vi "Temp Fuel Gen.vi"() -> ()   [LabVIEW 2017]
uses:
  Type defs/Control 1.ctl
panel:
  in  "f_q":dbl[][](array[numeric])
  in  "temp typedef":dbl[][](array[numeric])
  in  "Avg fuel 2":T1
  in  "output cluster 2":T1
  in  "Miliseconds to wait":dbl=1000.0 min=1000.0 step=1.0
  in  "Tryb auto":bool
  in  "Exit":bool
  in  "Wygeneruj":bool
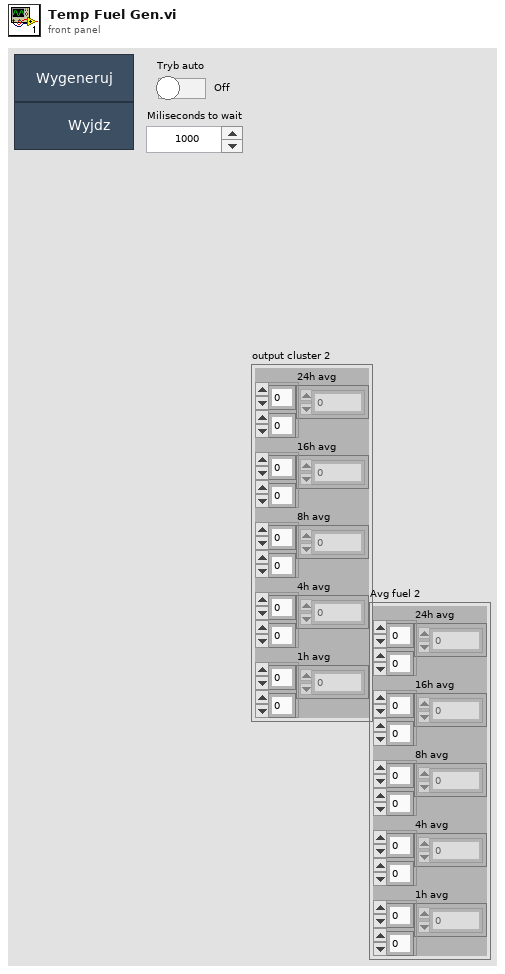
[diagram p1: front panel]
types:
  T1 = cluster{"24h avg":dbl[][], "16h avg":dbl[][], "8h avg":dbl[][], "4h avg":dbl[][], "1h avg":dbl[][]}
  T2 = typedef "Control 1.ctl" = enum16{"generate", "generate2", "wait for input", "timeout", "exit"}
  T3 = cluster{"Array":dbl[][], "Array":dbl[][], "Array":dbl[][], "Array":dbl[][], "Array":dbl[][]}
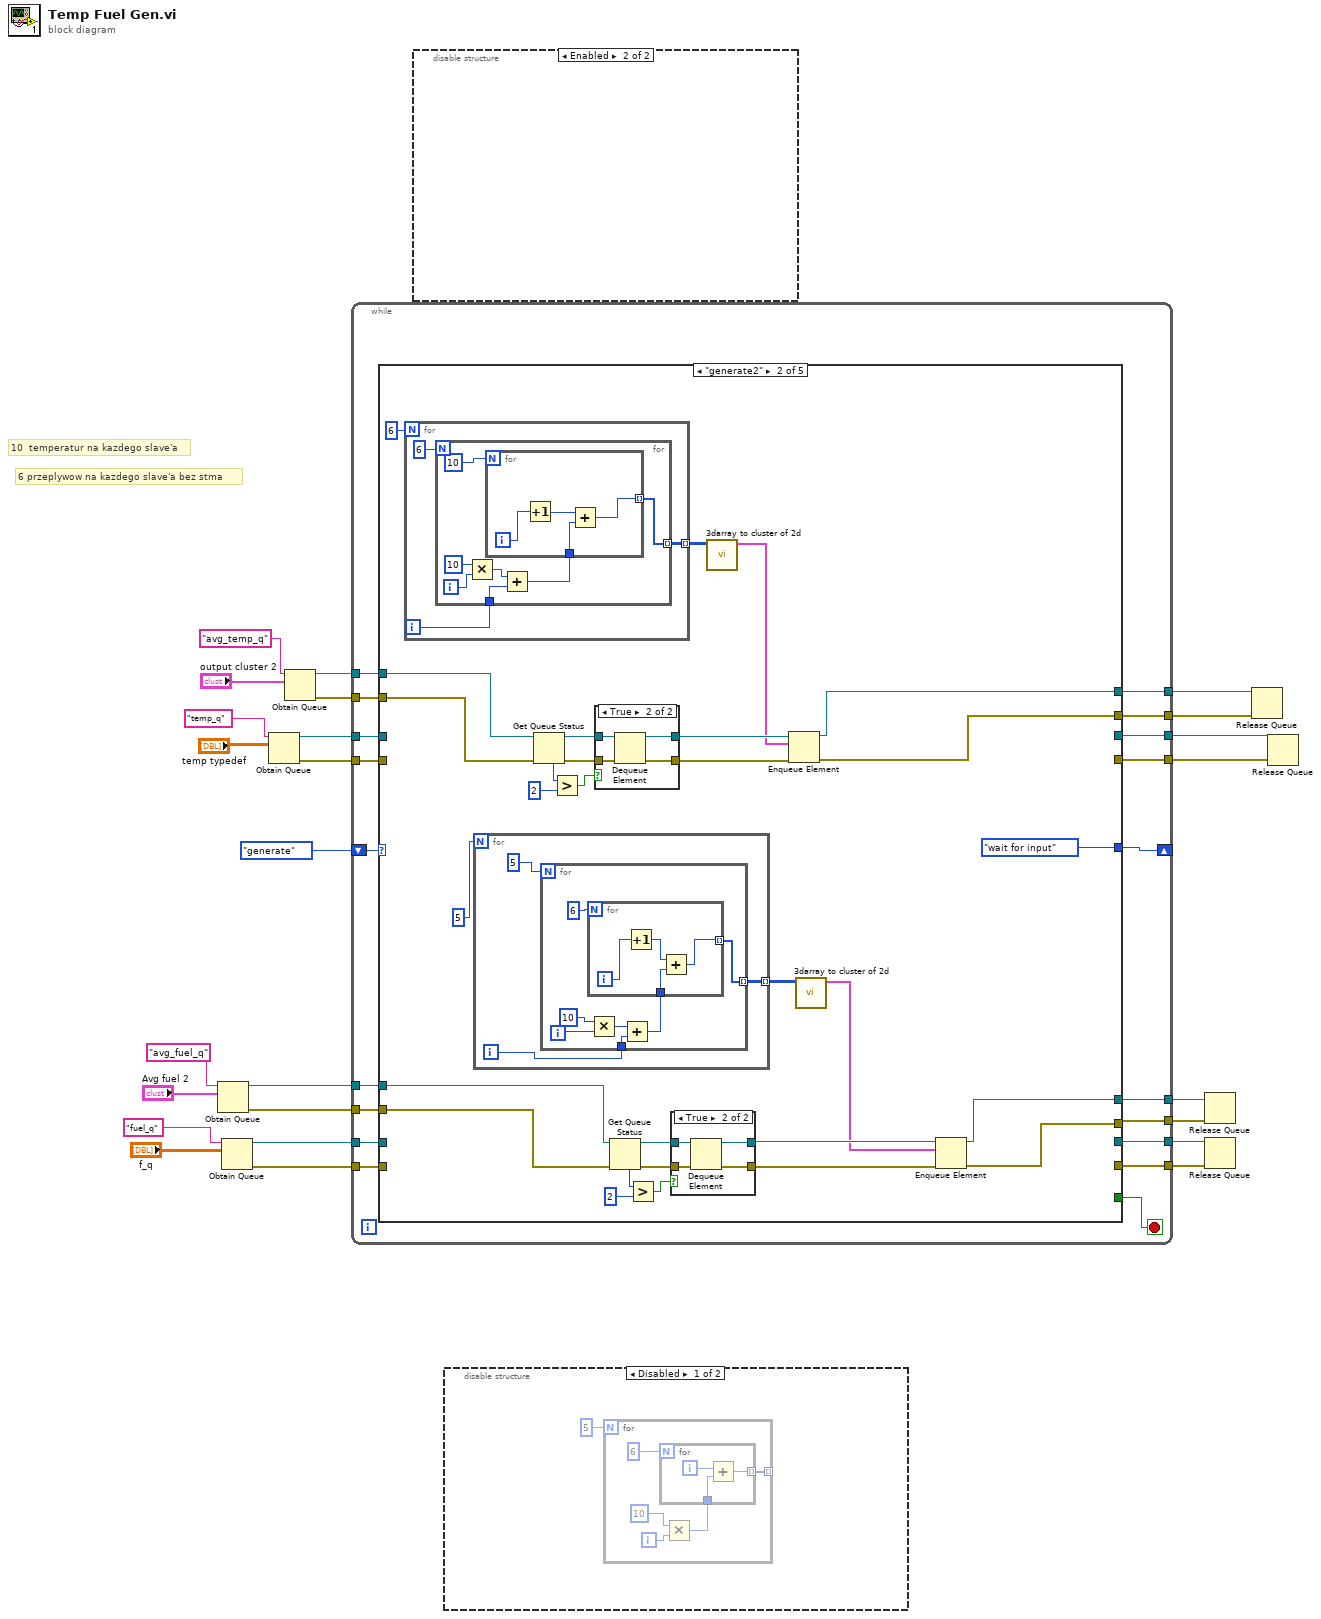
[diagram p0: block diagram]
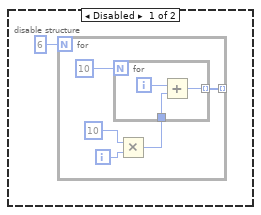
[diagram p3: hidden frame]
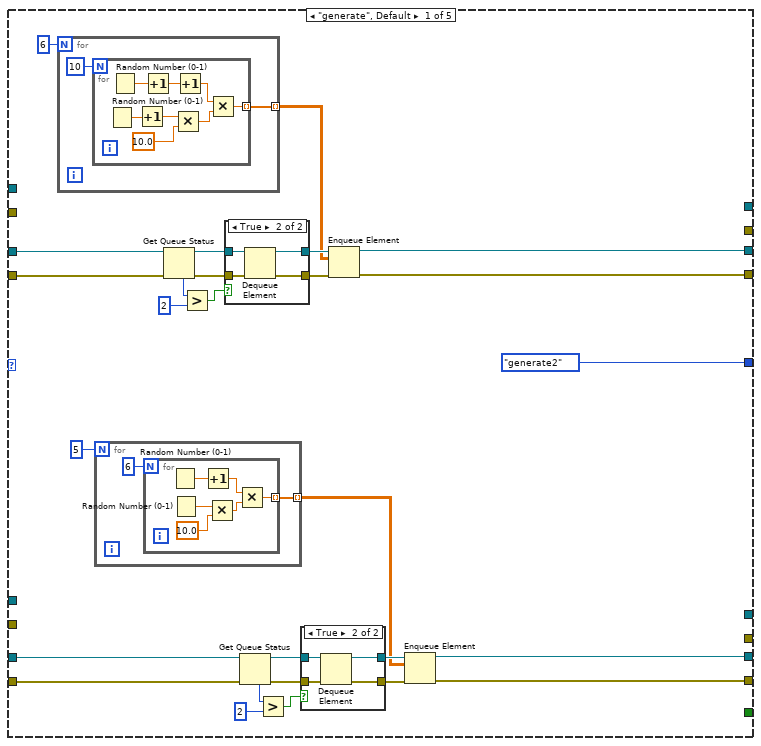
[diagram p4: hidden frame]
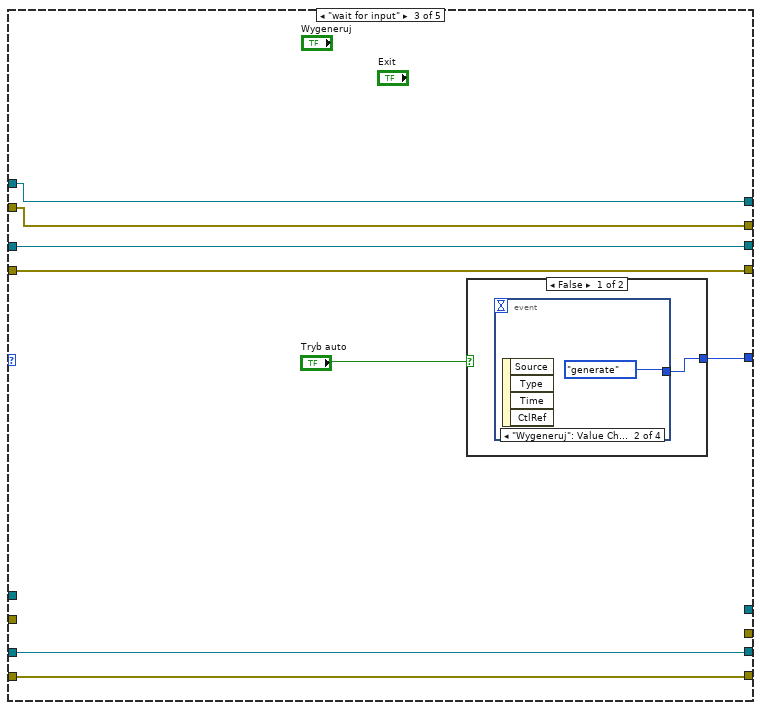
[diagram p9: hidden frame]
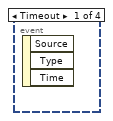
[diagram p10: hidden frame]
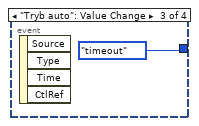
[diagram p11: hidden frame]
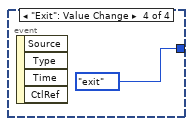
[diagram p12: hidden frame]
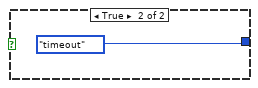
[diagram p13: hidden frame]
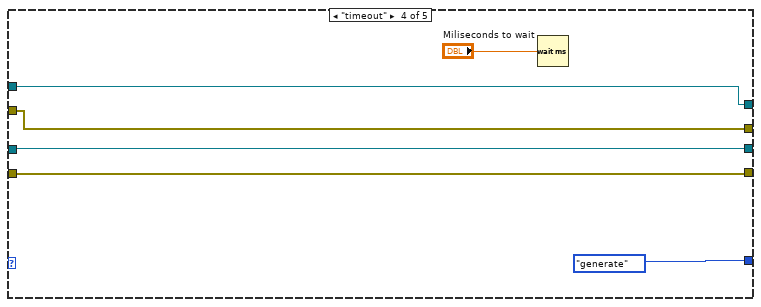
[diagram p14: hidden frame]
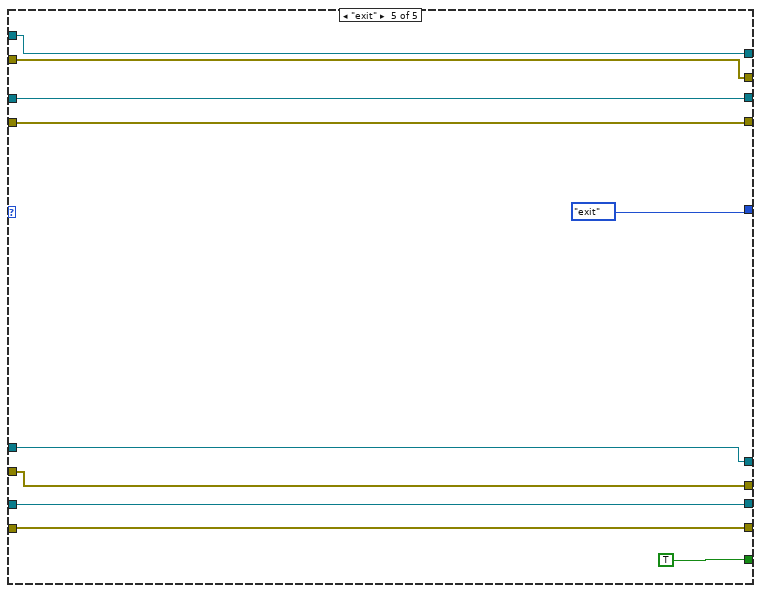
[diagram p15: hidden frame]
diagram:
  # "6 przeplywow na kazdego slave'a bez stma"
  # "10  temperatur na kazdego slave'a"
  n1 = Obtain Queue(name (unnamed)="avg_fuel_q", element data type="Avg fuel 2") -> (queue out=w7:refnum<queue>, error out=w8:errorcluster)  [unwired: 3 in, 1 out]
  n2 = Obtain Queue(name (unnamed)="fuel_q", element data type="f_q") -> (queue out=w21:refnum<queue>, error out=w20:errorcluster)  [unwired: 3 in, 1 out]
  n3 = Obtain Queue(name (unnamed)="temp_q", element data type="temp typedef") -> (queue out=w24:refnum<queue>, error out=w23:errorcluster)  [unwired: 3 in, 1 out]
  n4 = Obtain Queue(name (unnamed)="avg_temp_q", element data type="output cluster 2") -> (queue out=w5:refnum<queue>, error out=w6:errorcluster)  [unwired: 3 in, 1 out]
  n5 = while {
    tunnel: w24 -> [w44]
    tunnel: w23 -> [w43]
    tunnel: w21 -> [w42]
    tunnel: w20 -> [w41]
    tunnel: [w39] -> w19
    tunnel: [w38] -> w18
    tunnel: [w37] -> w17
    tunnel: [w36] -> w16
    shift-right: [w34] -> _
    shift-left: Control_1."generate" -> [w35]
    tunnel: w8 -> [w33]
    tunnel: w7 -> [w32]
    tunnel: w6 -> [w31]
    tunnel: w5 -> [w30]
    tunnel: [w29] -> w4
    tunnel: [w28] -> w3
    tunnel: [w27] -> w2
    tunnel: [w26] -> w1
    stop <- w40 stop-if-true
    n6 = case shown="\"generate2\"" w35 {
      tunnel: w44 -> [w64 _ w175 w185 w198]
      tunnel: w43 -> [w63 _ w174 w184 w197]
      tunnel: w42 -> [w55 _ w177 _ w196]
      tunnel: w41 -> [w54 _ w176 _ w195]
      tunnel: [Control_1."generate2" Control_1."wait for input" w178 Control_1."generate" Control_1."exit"] -> w34
      tunnel: [_ _ _ _ TRUE] -> w40
      tunnel: [w53 _ w175 w185 w198] -> w39
      tunnel: [w52 _ w174 w184 w197] -> w38
      tunnel: [w51 _ w177 _ w196] -> w37
      tunnel: [w50 _ w176 _ w195] -> w36
      tunnel: w33 -> [_ w114 _ _ w190]
      tunnel: w32 -> [_ w115 _ _ w191]
      tunnel: w31 -> [_ w112 w172 w186 w193]
      tunnel: w30 -> [_ w113 w171 w187 w192]
      tunnel: [_ w105 _ _ w191] -> w29
      tunnel: [_ w104 _ _ w190] -> w28
      tunnel: [_ w103 w171 w187 w192] -> w27
      tunnel: [_ w102 w172 w186 w193] -> w26
      frame "generate", Default {
        n7 = for {
          N: 6 -> [_]
          tunnel: [w80] -> w48 mode=indexing
          n8 = for {
            N: 10 -> [_]
            tunnel: [w82] -> w80 mode=indexing
            n9 = Random Number (0-1)() -> (number: 0 to 1=w86:dbl)
            n10 = Random Number (0-1)() -> (number: 0 to 1=w89:dbl)
            n11 = Increment(x=w86) -> (x+1=w85:dbl)
            n12 = Increment(x=w89) -> (x+1=w88:dbl)
            n13 = Multiply(x=w85, y=10.0) -> (x*y=w83:dbl)
            n14 = Increment(x=w88) -> (x+1=w87:dbl)
            n15 = Multiply(x=w87, y=w83) -> (x*y=w82:dbl)
          }
        }
        n16 = for {
          N: 5 -> [_]
          tunnel: [w72] -> w46 mode=indexing
          n17 = for {
            N: 6 -> [_]
            tunnel: [w76] -> w72 mode=indexing
            n18 = Random Number (0-1)() -> (number: 0 to 1=w79:dbl)
            n19 = Random Number (0-1)() -> (number: 0 to 1=w75:dbl)
            n20 = Increment(x=w79) -> (x+1=w74:dbl)
            n21 = Multiply(x=w75, y=10.0) -> (x*y=w77:dbl)
            n22 = Multiply(x=w74, y=w77) -> (x*y=w76:dbl)
          }
        }
        n23 = Get Queue Status(queue=w64, error in (no error)=w63) -> (queue out=w68:refnum<queue>, error out=w71:errorcluster, # elements in queue=w70:i32)  [unwired: 1 in, 5 out]
        n24 = Greater?(x=w70, y=2) -> (0:w67:bool)
        n25 = case shown="True" w67 {
          tunnel: w71 -> [w96 w101]
          tunnel: w68 -> [w97 w100]
          tunnel: [w97 w99] -> w66
          tunnel: [w96 w98] -> w65
          frame False {
          }
          frame True {
            n26 = Dequeue Element(queue=w100, error in (no error)=w101) -> (queue out=w99:refnum<queue>, error out=w98:errorcluster)  [unwired: 1 in, 2 out]
          }
        }
        n27 = Get Queue Status(queue=w55, error in (no error)=w54) -> (queue out=w59:refnum<queue>, error out=w61:errorcluster, # elements in queue=w60:i32)  [unwired: 1 in, 5 out]
        n28 = Greater?(x=w60, y=2) -> (0:w58:bool)
        n29 = case shown="True" w58 {
          tunnel: w61 -> [w90 w95]
          tunnel: w59 -> [w91 w94]
          tunnel: [w91 w93] -> w57
          tunnel: [w90 w92] -> w56
          frame False {
          }
          frame True {
            n30 = Dequeue Element(queue=w94, error in (no error)=w95) -> (queue out=w93:refnum<queue>, error out=w92:errorcluster)  [unwired: 1 in, 2 out]
          }
        }
        n31 = Enqueue Element(queue=w66, element=w48, error in (no error)=w65) -> (queue out=w53:refnum<queue>, error out=w52:errorcluster)  [unwired: 1 in, 1 out]
        n32 = Enqueue Element(queue=w57, element=w46, error in (no error)=w56) -> (queue out=w51:refnum<queue>, error out=w50:errorcluster)  [unwired: 1 in, 1 out]
      }
      frame "generate2" {
        n33 = for {
          N: 6 -> [_]
          tunnel: [w146] -> w111 mode=indexing
          i -> [w145]
          n34 = for {
            N: 6 -> [_]
            tunnel: [w153] -> w146 mode=indexing
            tunnel: w145 -> [w152]
            i -> [w151]
            n35 = Multiply(x=10, y=w151) -> (x*y=w149:i32)
            n36 = Add(x=w149, y=w152) -> (x+y=w148:i32)
            n37 = for {
              N: 10 -> [_]
              tunnel: [w155] -> w153 mode=indexing
              tunnel: w148 -> [w156]
              i -> [w158]
              n38 = Increment(x=w158) -> (x+1=w157:i32)
              n39 = Add(x=w157, y=w156) -> (x+y=w155:i32)
            }
          }
        }
        n40 = for {
          N: 5 -> [_]
          tunnel: [w132] -> w108 mode=indexing
          i -> [w131]
          n41 = for {
            N: 5 -> [_]
            tunnel: [w139] -> w132 mode=indexing
            tunnel: w131 -> [w135]
            i -> [w137]
            n42 = Multiply(x=10, y=w137) -> (x*y=w136:i32)
            n43 = Add(x=w136, y=w135) -> (x+y=w134:i32)
            n44 = for {
              N: 6 -> [_]
              tunnel: [w141] -> w139 mode=indexing
              tunnel: w134 -> [w142]
              i -> [w144]
              n45 = Increment(x=w144) -> (x+1=w143:i32)
              n46 = Add(x=w143, y=w142) -> (x+y=w141:i32)
            }
          }
        }
        n47 = Get Queue Status(queue=w113, error in (no error)=w112) -> (queue out=w127:refnum<queue>, error out=w130:errorcluster, # elements in queue=w129:i32)  [unwired: 1 in, 5 out]
        n48 = Greater?(x=w129, y=2) -> (0:w126:bool)
        n49 = case shown="True" w126 {
          tunnel: w130 -> [w165 w170]
          tunnel: w127 -> [w166 w169]
          tunnel: [w166 w168] -> w125
          tunnel: [w165 w167] -> w124
          frame False {
          }
          frame True {
            n50 = Dequeue Element(queue=w169, error in (no error)=w170) -> (queue out=w168:refnum<queue>, error out=w167:errorcluster)  [unwired: 1 in, 2 out]
          }
        }
        n51 = Get Queue Status(queue=w115, error in (no error)=w114) -> (queue out=w120:refnum<queue>, error out=w122:errorcluster, # elements in queue=w121:i32)  [unwired: 1 in, 5 out]
        n52 = Greater?(x=w121, y=2) -> (0:w119:bool)
        n53 = case shown="True" w119 {
          tunnel: w122 -> [w159 w164]
          tunnel: w120 -> [w160 w163]
          tunnel: [w160 w162] -> w107
          tunnel: [w159 w161] -> w118
          frame False {
          }
          frame True {
            n54 = Dequeue Element(queue=w163, error in (no error)=w164) -> (queue out=w162:refnum<queue>, error out=w161:errorcluster)  [unwired: 1 in, 2 out]
          }
        }
        n55 = call "3darray to cluster of 2d.vi"("Array"=w111) -> ("Cluster"=w110:T3)  [unwired: 10 in]
        n56 = Enqueue Element(queue=w125, element=w110, error in (no error)=w124) -> (queue out=w103:refnum<queue>, error out=w102:errorcluster)  [unwired: 1 in, 1 out]
        n57 = call "3darray to cluster of 2d.vi"("Array"=w108) -> ("Cluster"=w106:T3)  [unwired: 10 in]
        n58 = Enqueue Element(queue=w107, element=w106, error in (no error)=w118) -> (queue out=w105:refnum<queue>, error out=w104:errorcluster)  [unwired: 1 in, 1 out]
      }
      frame "wait for input" {
        n59 = case shown="False" "Tryb auto" {
          tunnel: [w179 Control_1."timeout"] -> w178
          frame False {
            n60 = event shown="[1] \"Wygeneruj\": Value Change" {
              selector: _ -> [_ _ _ _]
              dyn-events: _ -> [_ _ _ _]
              timeout: _ -> [_ _ _ _]
              tunnel: [_ Control_1."generate" Control_1."timeout" Control_1."exit"] -> w179
              event Timeout {
                n61 = event-data() -> ()  [unwired: 1 in, 3 out]
              }
              event "Wygeneruj": Value Change {
                n62 = event-data() -> ()  [unwired: 1 in, 4 out]
              }
              event "Tryb auto": Value Change {
                n63 = event-data() -> ()  [unwired: 1 in, 4 out]
              }
              event "Exit": Value Change {
                n64 = event-data() -> ()  [unwired: 1 in, 4 out]
              }
            }
          }
          frame True {
          }
        }
      }
      frame "timeout" {
        n65 = Wait (ms)(milliseconds to wait="Miliseconds to wait") -> ()  [unwired: 1 out]
      }
      frame "exit" {
      }
    }
  }
  n66 = disable-structure shown="Enabled" {
    frame Disabled {
      n67 = for {
        N: 6 -> [_]
        tunnel: [w201] -> _ mode=indexing
        i -> [w204]
        n68 = Multiply(x=10, y=w204) -> (x*y=w202:i32)
        n69 = for {
          N: 10 -> [_]
          tunnel: w202 -> [w207]
          tunnel: [w206] -> w201 mode=indexing
          i -> [w208]
          n70 = Add(x=w208, y=w207) -> (x+y=w206:i32)
        }
      }
    }
    frame Enabled {
    }
  }
  n71 = disable-structure shown="Disabled" {
    frame Disabled {
      n72 = for {
        N: 5 -> [_]
        tunnel: [w210] -> _ mode=indexing
        i -> [w213]
        n73 = Multiply(x=10, y=w213) -> (x*y=w211:i32)
        n74 = for {
          N: 6 -> [_]
          tunnel: w211 -> [w216]
          tunnel: [w215] -> w210 mode=indexing
          i -> [w217]
          n75 = Add(x=w217, y=w216) -> (x+y=w215:i32)
        }
      }
    }
    frame Enabled {
    }
  }
  n76 = Release Queue(queue=w4, error in (no error)=w3) -> ()  [unwired: 1 in, 3 out]
  n77 = Release Queue(queue=w17, error in (no error)=w16) -> ()  [unwired: 1 in, 3 out]
  n78 = Release Queue(queue=w2, error in (no error)=w1) -> ()  [unwired: 1 in, 3 out]
  n79 = Release Queue(queue=w19, error in (no error)=w18) -> ()  [unwired: 1 in, 3 out]
